vi "Fill with Zero.vi"(8 "Nbre caractères":u8, 11 "String IN":string) -> (3 "String OUT":string)   [LabVIEW 2020, in "Exaprom PDF.lvlib"]
uses:
  <userlib>/labview-PDF-writer-master/Exaprom PDF.lvlib
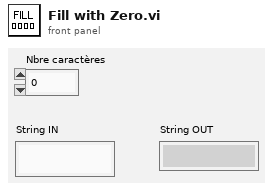
[diagram p1: front panel]
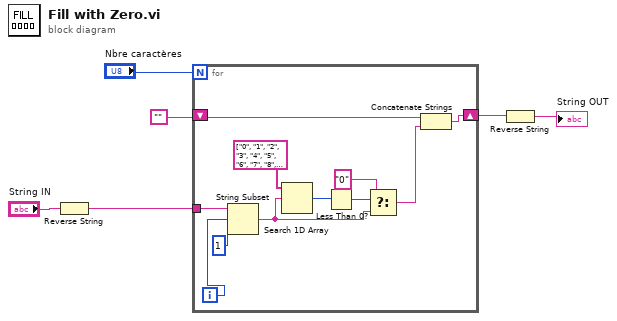
[diagram p0: block diagram]
diagram:
  n1 = Reverse String(1:"String IN") -> (0:w4:string)
  n2 = for {
    N: "Nbre caractères" -> [_]
    tunnel: w4 -> [w17]
    shift-right: [w9] -> w2
    shift-left: "" -> [w8]
    i -> [w16]
    n3 = String Subset(string=w17, offset (0)=w16, length (rest)=1 ("length (rest)")) -> (substring=w11:string)
    n4 = Search 1D Array(1D array=string[] ["0", "1", "2", "3", "4", "5", "6", "7", "8", "9"], element=w11) -> (index of element=w13:i32)  [unwired: 1 out]
    n5 = Less Than 0?(x=w13) -> (x < 0?=w12:bool)
    n6 = Select(t="0", s=w12, f=w11) -> (s? t:f=w7:string)
    n7 = Concatenate Strings(w8, w7) -> (w9:string)
  }
  n8 = Reverse String(1:w2) -> (0:→"String OUT":string)
